vi "SetMenuState.vi"(10 "Authorization":string, 11 "Menu":refnum<k9>) -> ()   [LabVIEW 2014]
doc: "Sets all the controls in the input array to the \"Enable state\" value."
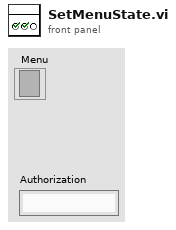
[diagram p1: front panel]
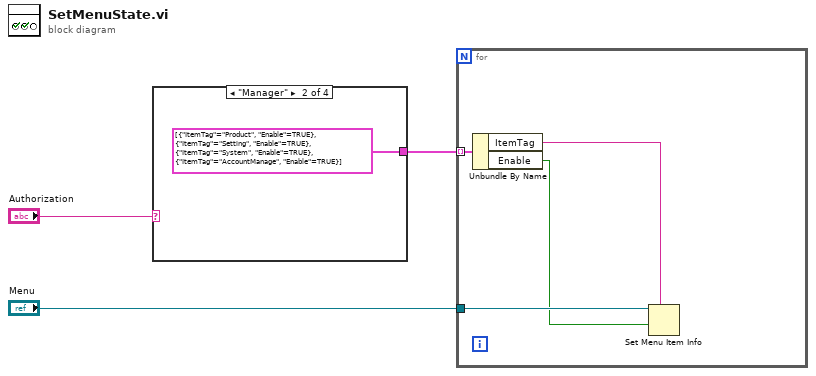
[diagram p0: block diagram]
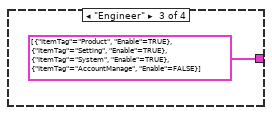
[diagram p3: hidden frame]
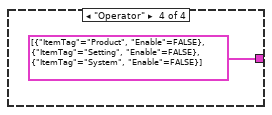
[diagram p4: hidden frame]
diagram:
  n1 = case shown="\"Manager\"" "Authorization" {
    tunnel: [_ cluster{"ItemTag":string, "Enable":bool}[] [{"ItemTag"="Product", "Enable"=TRUE}, {"ItemTag"="Setting", "Enable"=TRUE}, {"ItemTag"="System", "Enable"=TRUE}, {"ItemTag"="AccountManage", "Enable"=TRUE}] cluster{"ItemTag":string, "Enable":bool}[] [{"ItemTag"="Product", "Enable"=TRUE}, {"ItemTag"="Setting", "Enable"=TRUE}, {"ItemTag"="System", "Enable"=TRUE}, {"ItemTag"="AccountManage", "Enable"=FALSE}] cluster{"ItemTag":string, "Enable":bool}[] [{"ItemTag"="Product", "Enable"=FALSE}, {"ItemTag"="Setting", "Enable"=FALSE}, {"ItemTag"="System", "Enable"=FALSE}]] -> w1
    frame Default {
    }
    frame "Manager" {
    }
    frame "Engineer" {
    }
    frame "Operator" {
    }
  }
  n2 = for {
    tunnel: "Menu" -> [w10]
    tunnel: w1 -> [w9] mode=indexing
    n3 = Unbundle By Name(w9) -> ("ItemTag"=w8:string, "Enable"=w7:bool)
    n4 = Set Menu Item Info(7:w8, 9:w7, 11:w10) -> ()  [unwired: 4 in, 2 out]
  }
